vi "EjemploDSC.vi"() -> ()   [LabVIEW 2020]
panel:
  in  "Slide 2":dbl(slide) scale=0.0..10.0
  in  "Slide":dbl(slide) scale=0.0..10.0
  in  "stop":bool
  out "Boolean 2":bool
  in  "Boolean":bool
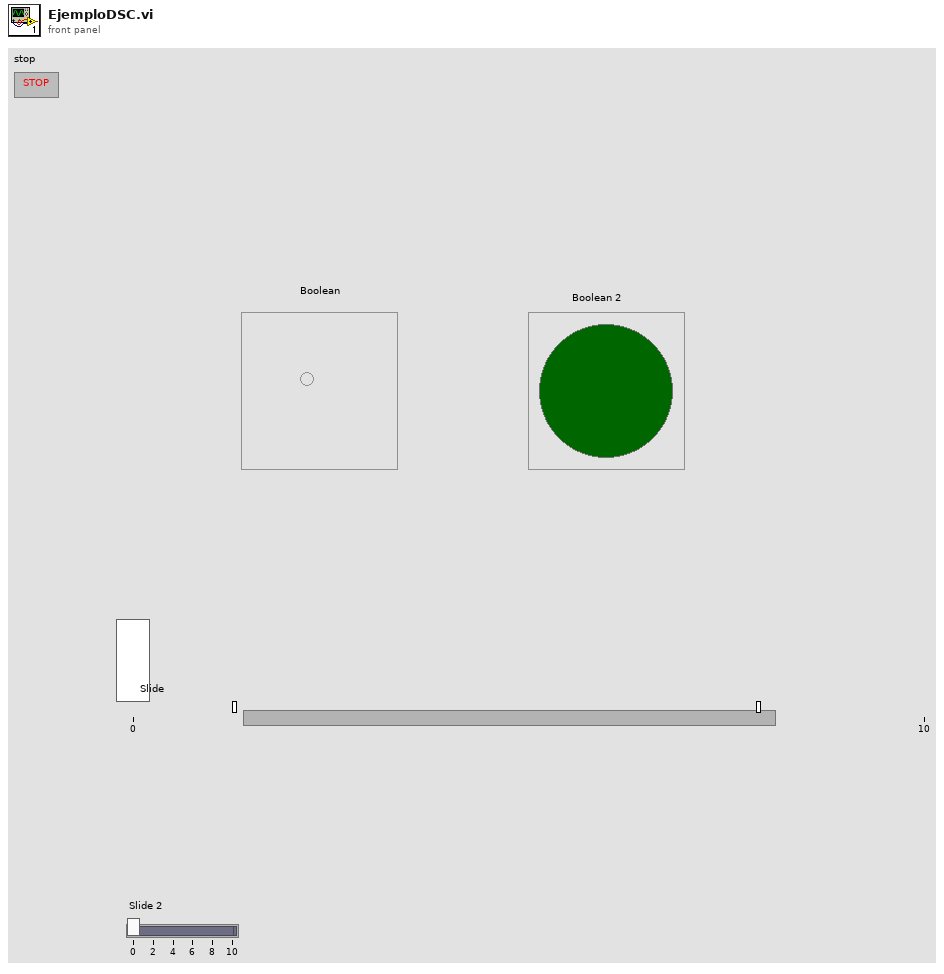
[diagram p1: front panel]
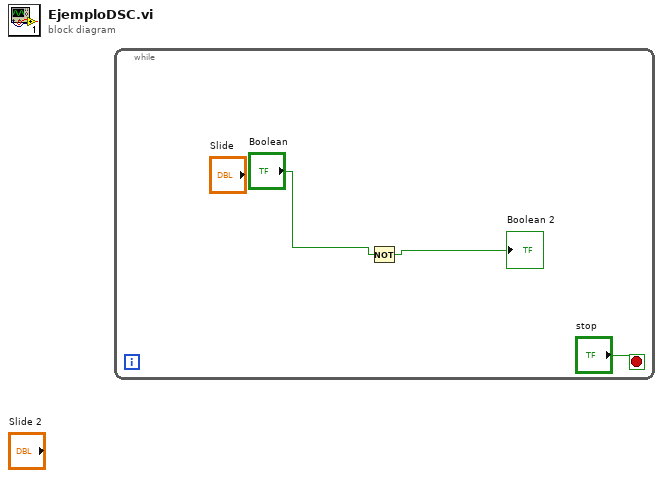
[diagram p0: block diagram]
diagram:
  n1 = while {
    stop <- "stop" stop-if-true
    n2 = Not(x="Boolean") -> (.not. x?=→"Boolean 2":bool)
  }
